vi "Set ni_measurementlink_measurement_v2_ConfigurationParameter_AnnotationsEntry.vi"(7 "Complete Call (T)":bool=TRUE, 8 "error in (no error)":errorcluster, 10 "package_templatemessage":T1, 11 "gRPCid":T2) -> (0 "error out":errorcluster)   [LabVIEW 2020, in "MeasurementLink Measurement Service Base V2.lvlib"]
uses:
  MeasurementLink Measurement Service Base V2.lvlib
  <vilib>/gRPC/LabVIEW gRPC Library/Shared/grpcId.ctl
  ni_measurementlink_measurement_v2_ConfigurationParameter_AnnotationsEntry.ctl
  dcc74a39-081a-4bdd-860b-8ed792803c96.vi
  <vilib>/gRPC/LabVIEW gRPC Library/Shared/TranslateGrpcError.vi
  <vilib>/gRPC/LabVIEW gRPC Library/Server API/Server/Get Server DLL Path.vi
  <vilib>/Utility/error.llb/Error Cluster From Error Code.vi
  <vilib>/gRPC/LabVIEW gRPC Library/grpc-lvsupport-release.lvlib
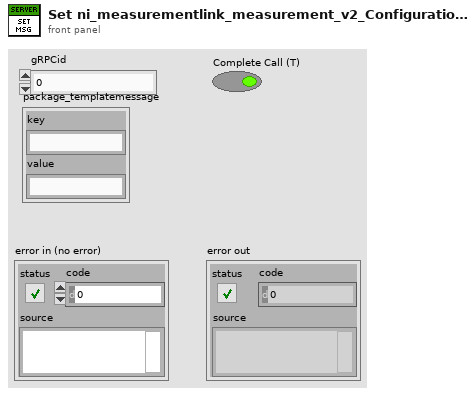
[diagram p1: front panel]
types:
  T1 = typedef "MeasurementLink Measurement Service Base V2.lvlib/ni_measurementlink_measurement_v2_ConfigurationParameter_AnnotationsEntry.ctl" = cluster{"key":string, "value":string}
  T2 = typedef "grpc-lvsupport-release.lvlib/grpcId.ctl" = u64
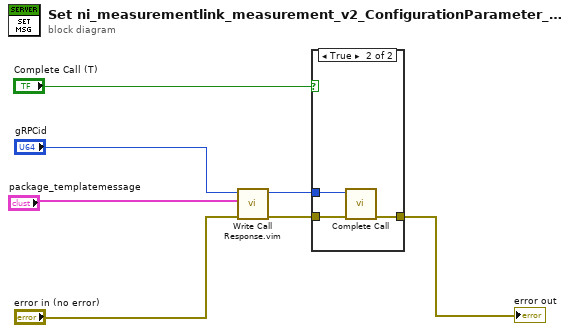
[diagram p0: block diagram]
diagram:
  n1 = call "Write Call Response.vim"("error in"="error in (no error)", "Response Data"="package_templatemessage", "gRPCid in"="gRPCid") -> ("error out"=w4:errorcluster, "gRPCid out"=w5:T2)  [unwired: 7 in]
  n2 = case shown="True" "Complete Call (T)" {
    tunnel: [w8 w11] -> w7
    tunnel: w5 -> [_ w10]
    tunnel: w4 -> [w8 w9]
    frame False {
    }
    frame True {
      n3 = call <vilib>:"Complete Call.vi"("gRPCid"=w10, "error in"=w9) -> ("error out"=w11:errorcluster)  [unwired: 8 in]
    }
  }
  "error out" <- w7
